vi "F Dwf Digital In Status Noise2.vi"(7 "countOfDataBytes":i32, 8 "error in (no error)":errorcluster, 9 "idxSample":i32, 10 "rgData":u32, 11 "hdwf":i32) -> (0 "error out":errorcluster, 2 "rgData out":u32, 3 "function return":i32)   [LabVIEW 2019, in "Olasdwf.lvlib"]
doc: "DWFAPI int FDwfDigitalInStatusNoise2(HDWF hdwf, void *rgData, int idxSample, int countOfDataBytes);"
uses:
  Olasdwf.lvlib
  Windows/System32/dwf.dll
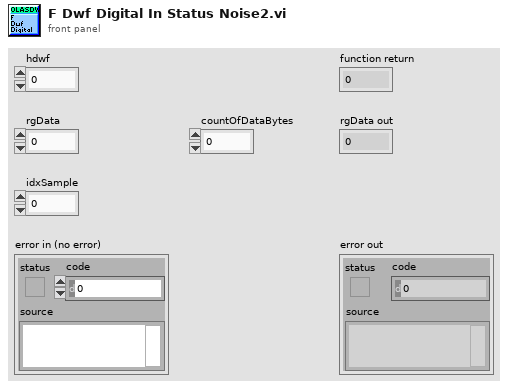
[diagram p1: front panel]
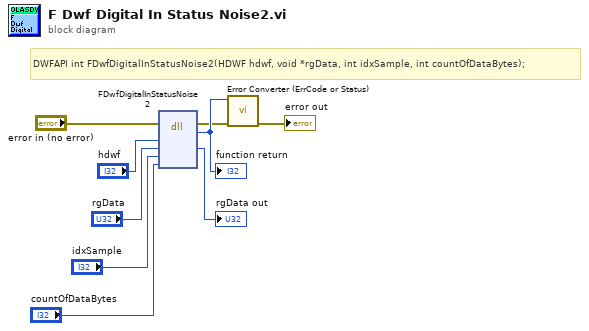
[diagram p0: block diagram]
diagram:
  # "DWFAPI int FDwfDigitalInStatusNoise2(HDWF hdwf, void *rgData, int idxSample, int countOfDataBytes);"
  n1 = dll-call lib="C:/Windows/System32/dwf.*" fn="FDwfDigitalInStatusNoise2"(error in="error in (no error)", "hdwf"="hdwf", "rgData"="rgData", "idxSample"="idxSample", "countOfDataBytes"="countOfDataBytes") -> (error out=w2:errorcluster, w9:i32, "rgData"=→"rgData out":u32)  [unwired: 5 in, 1 out]
  "function return" <- w9
  n2 = call "Error Converter (ErrCode or Status).vi"("error in (no error)"=w2, "error code"=w9) -> ("error out"=→"error out":errorcluster)  [unwired: 9 in]
